vi "user initialization.vi"(8 "error in":errorcluster, 10 "configuration in":refnum<class "control module configuration.lvclass">, 11 "fixed channel runtime in":refnum<class "MotionModule runtime.lvclass">) -> (0 "error out":errorcluster, 3 "fixed channel runtime out":refnum<class "MotionModule runtime.lvclass">)   [LabVIEW 2017, in "MotionModule runtime.lvclass"]
uses:
  MotionModule runtime.lvclass
  <vilib>/NI/DCAF/Tag Editor Core/control module/configuration/control module configuration.lvclass
  configuration/MotionModule configuration.lvclass
  <vilib>/NI/DCAF/Tag Editor Core/control module/runtime/control module runtime.lvclass
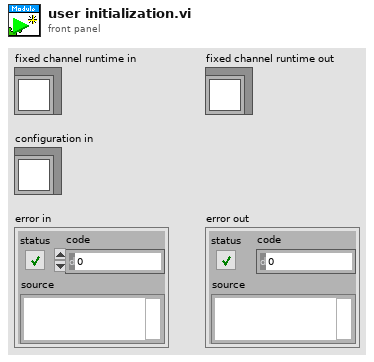
[diagram p1: front panel]
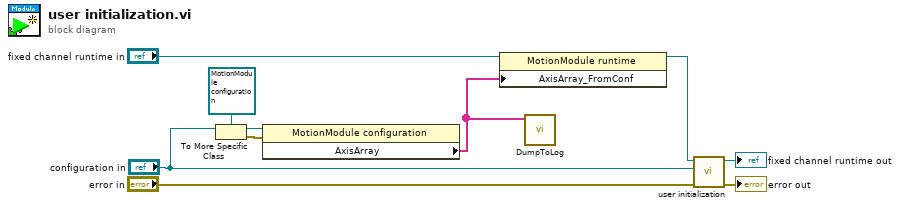
[diagram p0: block diagram]
diagram:
  n1 = To More Specific Class(target class=refnum<class "MotionModule configuration.lvclass"> refnum ("MotionModule configuration"), reference="configuration in") -> (specific class reference=w4:refnum<class "MotionModule configuration.lvclass">, error out=w1:errorcluster)  [unwired: 1 in]
  n2 = property class="MotionModule configuration"(reference=w4, error in=w1) -> ("AxisArray"=w2:string[])  [unwired: 2 out]
  n3 = property class="MotionModule runtime"(reference="fixed channel runtime in", "AxisArray_FromConf"=w2) -> (reference out=w6:refnum<class "MotionModule runtime.lvclass">)  [unwired: 1 in, 1 out]
  n4 = call "DumpToLog.vi"("DataToLog"=w2) -> ()  [unwired: 11 in]
  n5 = call-parent "user initialization.vi"("error in"="error in", "configuration in"="configuration in", "fixed channel runtime in"=w6) -> ("error out"=→"error out":errorcluster, "fixed channel runtime out"=→"fixed channel runtime out":refnum<class "MotionModule runtime.lvclass">)  [unwired: 7 in]
